vi "Goal Picker.vi"(6 "ResolutionX":dbl, 10 "InArray":dbl[][](array[numeric])) -> (3 "SelectedGoalSubarray":dbl[](array[numeric]))   [LabVIEW 2012]
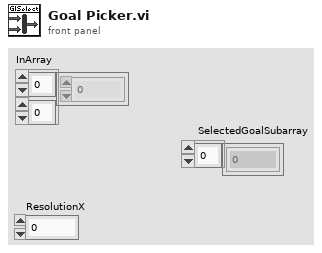
[diagram p1: front panel]
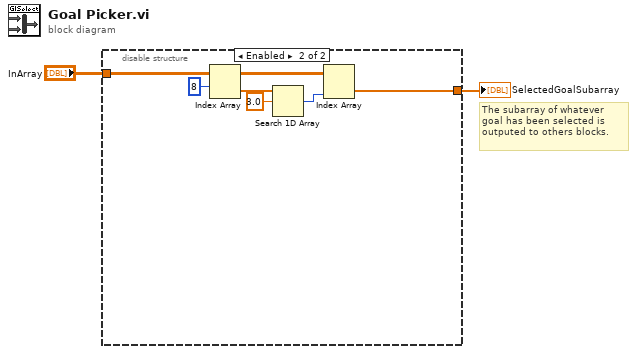
[diagram p0: block diagram]
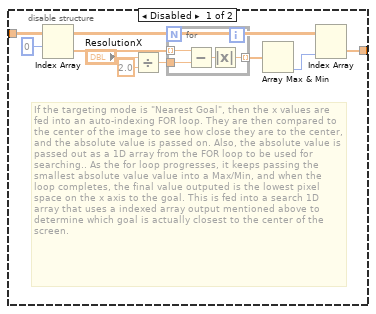
[diagram p2: hidden frame]
diagram:
  # "The subarray of whatever goal has been selected is outputed to others blocks."
  n1 = disable-structure shown="Enabled" {
    disable-tunnel: "InArray" -> [w11 w18]
    disable-tunnel: [w10 w17] -> w1
    frame Disabled {
      # "If the targeting mode is \"Nearest Goal\", then the x values are fed into an auto-indexing FOR loop. They are then compared to the center of the image to see how close they are to the center, and the absolute value is passed on. Also, the absolute value is passed out as a 1D array from the FOR loop to be used for searching.. As the for loop progresses, it keeps passing the smallest absolute value value into a Max/Min, and when the loop completes, the final value outputed is the lowest pixel space on the x axis to the goal. This is fed into a search 1D array that uses a indexed array output mentioned above to determine which goal is actually closest to the center of the screen."
      n2 = Index Array(array=w11, index (row)=0) -> (element=w5:dbl[])  [unwired: 1 in]
      n3 = Divide(x="ResolutionX", y=2.0) -> (x/y=w7:dbl)
      n4 = for {
        tunnel: w5 -> [w15] mode=indexing
        tunnel: w7 -> [w13]
        tunnel: [w12] -> w4 mode=indexing
        n5 = Subtract(x=w15, y=w13) -> (x-y=w14:dbl)
        n6 = Absolute Value(x=w14) -> (abs(x)=w12:dbl)
      }
      n7 = Array Max & Min(array=w4) -> (min index (indices)=w3:i32)  [unwired: 3 out]
      n8 = Index Array(array=w11, index (col)=w3) -> (element=w10:dbl[])  [unwired: 1 in]
    }
    frame Enabled {
      n9 = Index Array(array=w18, index (row)=8) -> (element=w20:dbl[])  [unwired: 1 in]
      n10 = Search 1D Array(1D array=w20, element=3.0) -> (index of element=w16:i32)  [unwired: 1 in]
      n11 = Index Array(array=w18, index (col)=w16) -> (element=w17:dbl[])  [unwired: 1 in]
    }
  }
  "SelectedGoalSubarray" <- w1
